vi "XIPIN_AXI_USB2_Device_5_0.vi"   [LabVIEW 2017]
doc: "USB2.0 end point device\n------------------------------------\n<b>Need License</b> : Yes\n<b>Interface</b> : AXI4"
uses:
  <vilib>/rvi/XilinxIP/XIPIN_XNode/niFpgaXIPIN.xnode
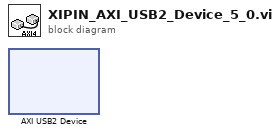
[diagram p0: block diagram]
diagram:
  n1 = xnode ("AXI USB2 Device")() -> ()
